vi "Text to UTF-8.vi"   [LabVIEW 2020, in "G-Unicode.lvlib"]
uses:
  G-Unicode.lvlib
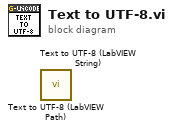
[diagram p0: block diagram]
diagram:
  n1 = call "Text to UTF-8 (LabVIEW Path).vi"() -> ()  [unwired: 10 in, 2 out]
  n2 = call "Text to UTF-8 (LabVIEW String).vi"() -> ()  [unwired: 10 in, 2 out]
